vi "CounterToRad.vi"(11 "Counter Value":i32) -> (3 "rads":dbl)   [LabVIEW 2019]
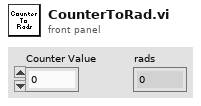
[diagram p1: front panel]
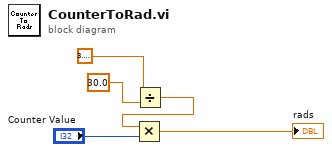
[diagram p0: block diagram]
diagram:
  n1 = Divide(x=3.141592653589793, y=30.0) -> (x/y=w4:dbl)
  n2 = Multiply(x=w4, y="Counter Value") -> (x*y=→"rads":dbl)
